vi "Red-Blue Overlay with Select.vi"(7 "RGB IMageRefnum IN":T1, 8 "Blue Channel Refnum":T1, 9 "Enable Blue?":bool, 10 "Red Channel Refnum":T1, 11 "Enable Red?":bool) -> (3 "RGB Image Refnum out OUT":T1)   [LabVIEW 2012]
uses:
  <vilib>/vision/Image Controls.llb/IMAQ Image.ctl
  <vilib>/vision/NI_Vision_Development_Module.lvlib
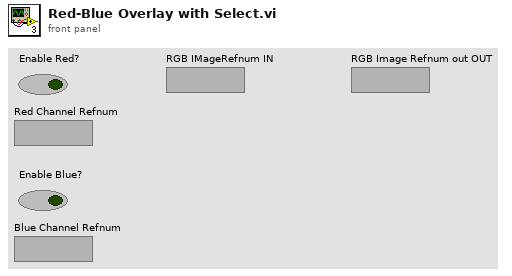
[diagram p1: front panel]
types:
  T1 = typedef "IMAQ Image.ctl" = refnum<image>
  T2 = typedef "Image Type" = u32
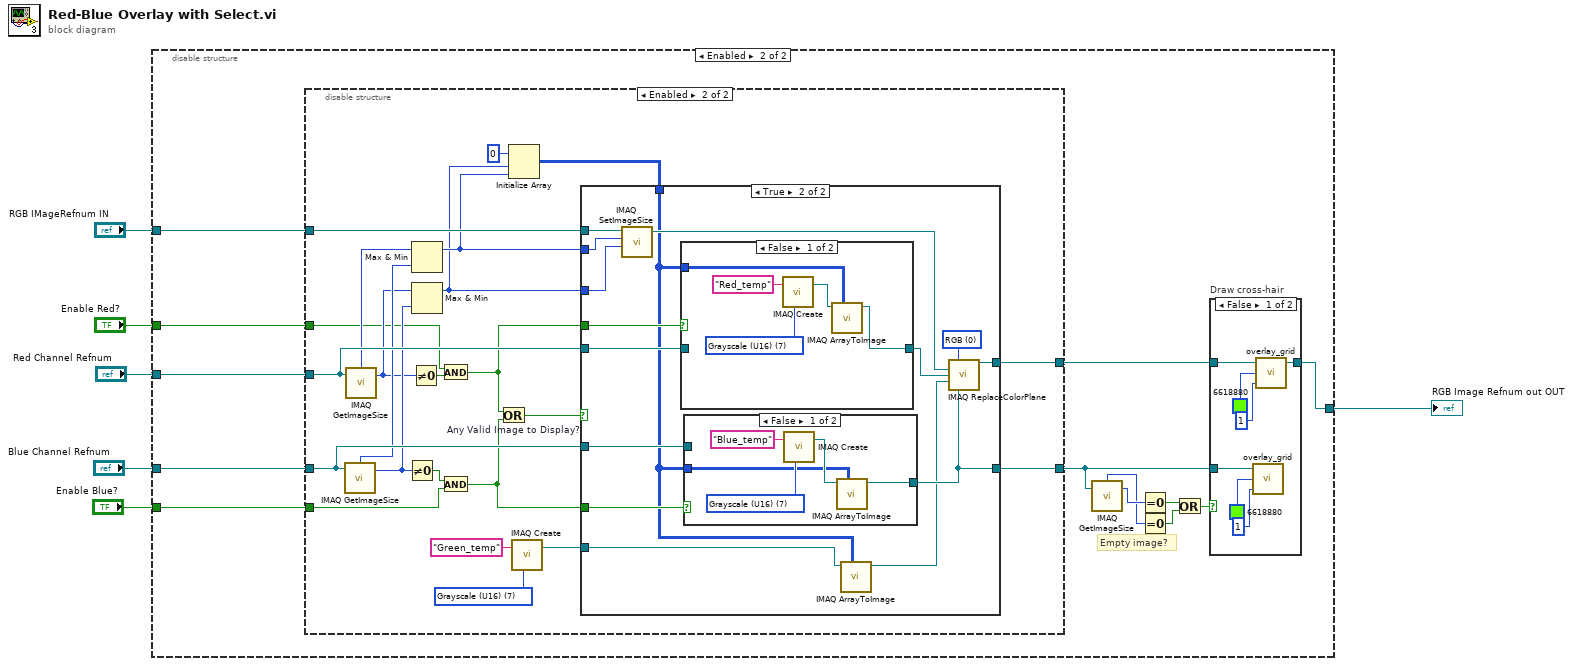
[diagram p0: block diagram]
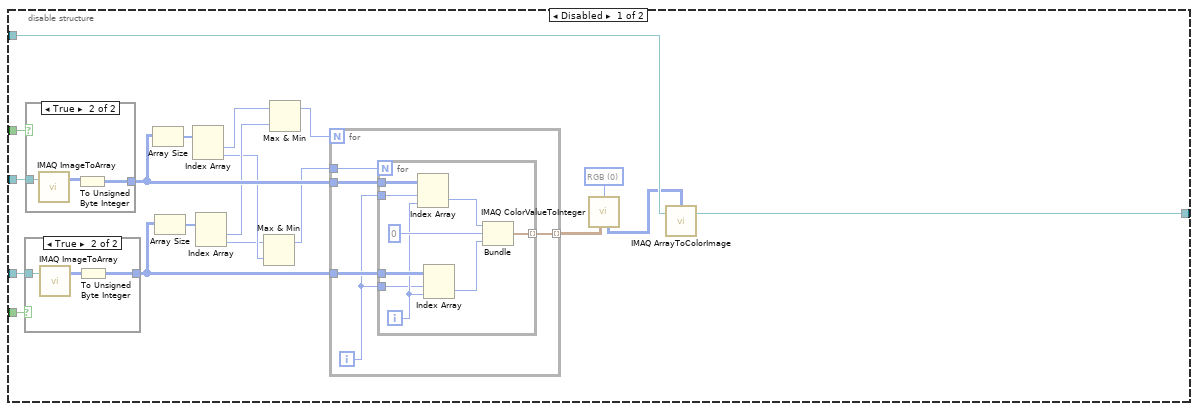
[diagram p2: hidden frame]
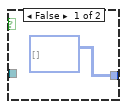
[diagram p3: hidden frame]
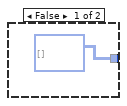
[diagram p4: hidden frame]
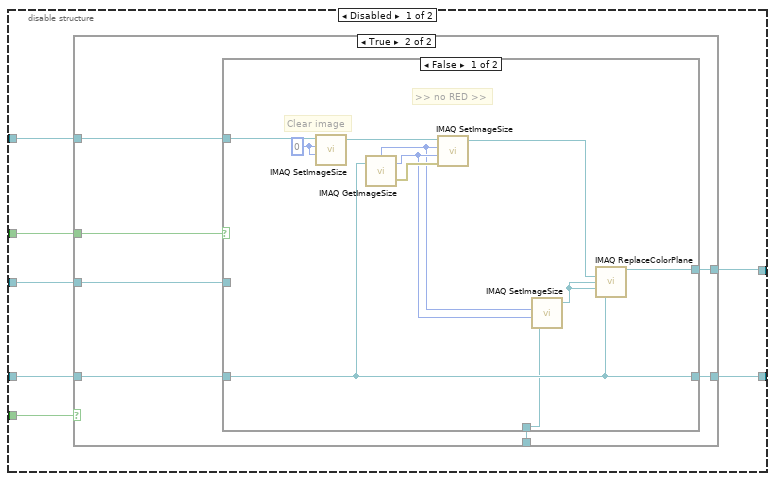
[diagram p5: hidden frame]
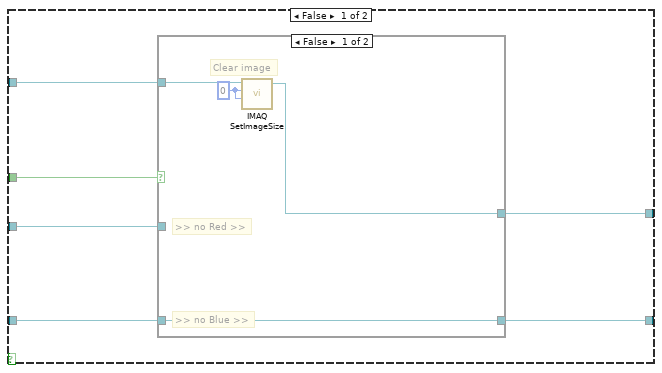
[diagram p6: hidden frame]
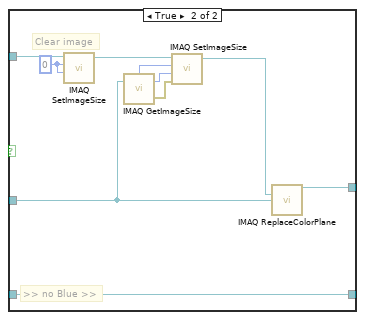
[diagram p7: hidden frame]
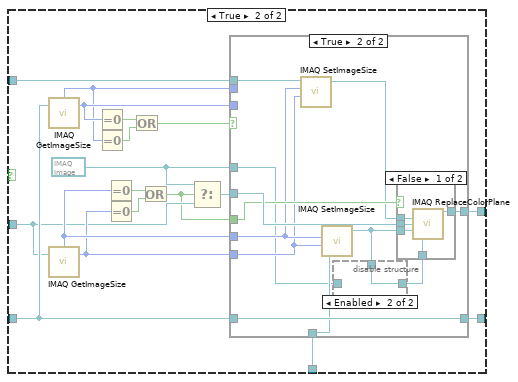
[diagram p8: hidden frame]
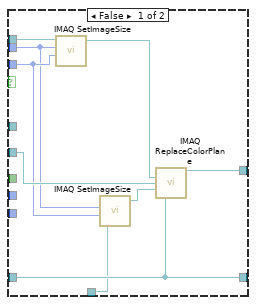
[diagram p9: hidden frame]
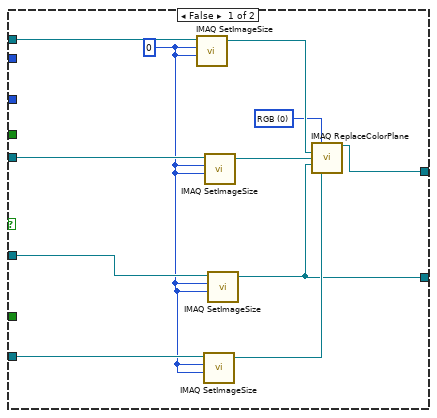
[diagram p12: hidden frame]
diagram:
  n1 = disable-structure shown="Enabled" {
    disable-tunnel: [w25 w48] -> w1
    disable-tunnel: "Blue Channel Refnum" -> [w23 w57]
    disable-tunnel: "Red Channel Refnum" -> [w22 w58]
    disable-tunnel: "RGB IMageRefnum IN" -> [w21 w56]
    disable-tunnel: "Enable Blue?" -> [w18 w59]
    disable-tunnel: "Enable Red?" -> [w17 w60]
    frame Disabled {
      w20 = u16 0 items=["RGB", "HSL", "HSV", "HSI"] ("Color Mode")
      n2 = case shown="True" w18 {
        tunnel: [u8[][] [] w33] -> w16
        tunnel: w23 -> [_ w31]
        frame False {
        }
        frame True {
          n3 = call "IMAQ ImageToArray"("Image"=w31) -> ("Image Pixels (I16)"=w32:i16[][])  [unwired: 3 in, 4 out]
          n4 = To Unsigned Byte Integer(number=w32) -> (unsigned 8bit integer=w33:u8[][])
        }
      }
      n5 = case shown="True" w17 {
        tunnel: [u8[][] [] w29] -> w15
        tunnel: w22 -> [_ w27]
        frame False {
        }
        frame True {
          n6 = call "IMAQ ImageToArray"("Image"=w27) -> ("Image Pixels (I16)"=w28:i16[][])  [unwired: 3 in, 4 out]
          n7 = To Unsigned Byte Integer(number=w28) -> (unsigned 8bit integer=w29:u8[][])
        }
      }
      n8 = Array Size(array=w15) -> (size(s)=w14:i32[])
      n9 = Array Size(array=w16) -> (size(s)=w13:i32[])
      n10 = Index Array(array=w14) -> (element #1=w12:i32, element #2=w9:i32)  [unwired: 2 in]
      n11 = Index Array(array=w13) -> (element #1=w10:i32, element #2=w7:i32)  [unwired: 2 in]
      n12 = Max & Min(x=w7, y=w9) -> (max(x,y)=w8:i32)  [unwired: 1 out]
      n13 = Max & Min(x=w12, y=w10) -> (max(x,y)=w11:i32)  [unwired: 1 out]
      n14 = for {
        N: w11 -> [_]
        tunnel: w16 -> [w35]
        tunnel: w15 -> [w38]
        tunnel: [w37] -> w24 mode=indexing
        tunnel: w8 -> [w36]
        i -> [w34]
        n15 = for {
          N: w36 -> [_]
          tunnel: w38 -> [w44]
          tunnel: [w46] -> w37 mode=indexing
          tunnel: w35 -> [w45]
          tunnel: w34 -> [w42]
          tunnel: w34 -> [w41]
          i -> [w43]
          n16 = Index Array(array=w44, index (row)=w41, index (col)=w43) -> (element=w40:u8)
          n17 = Index Array(array=w45, index (row)=w42, index (col)=w43) -> (element=w39:u8)
          n18 = Bundle(w40, u8 0, w39) -> (w46:cluster{u8, u8, u8})  [unwired: 1 in]
        }
      }
      n19 = call "IMAQ ColorValueToInteger"("2D Color value array"=w24, "Color Mode"=w20) -> ("2D U32 array"=w19:u32[][])  [unwired: 3 in, 3 out]
      n20 = call "IMAQ ArrayToColorImage"("Image Pixels (U32)"=w19, "Image"=w21) -> ("Image Out"=w25:T1)  [unwired: 3 in, 1 out]
    }
    frame Enabled {
      # "Empty image?"
      n21 = disable-structure shown="Enabled" {
        disable-tunnel: w60 -> [w68 w167]
        disable-tunnel: w59 -> [w67 w169]
        disable-tunnel: w58 -> [w66 w175]
        disable-tunnel: w57 -> [w65 w176]
        disable-tunnel: w56 -> [w64 w165]
        disable-tunnel: [w63 w163] -> w52
        disable-tunnel: [w62 w164] -> w49
        frame Disabled {
          n22 = case shown="True" w67 {
            tunnel: w64 -> [w73 w95]
            tunnel: w66 -> [w72 w94]
            tunnel: [w70 w93] -> w62
            tunnel: w68 -> [w74 w92]
            tunnel: w65 -> [w71 w91]
            tunnel: [w69 w90] -> w63
            tunnel: [_ w89] -> w61
            frame False {
              n23 = case shown="False" w74 {
                tunnel: [w76 w88] -> w70
                tunnel: w73 -> [w77 w82]
                tunnel: w72 -> [_ w84]
                tunnel: w71 -> [w75 w80]
                tunnel: [w75 w80] -> w69
                frame False {
                  w78 = 0 ("X Resolution")
                  # "Clear image"
                  # ">> no Blue >>"
                  # ">> no Red >>"
                  n24 = call "IMAQ SetImageSize"("Y Resolution"=w78, "X Resolution"=w78, "Image"=w77) -> ("Image Out"=w76:T1)  [unwired: 2 in, 1 out]
                }
                frame True {
                  w83 = 0 ("X Resolution")
                  # "Clear image"
                  # ">> no Blue >>"
                  n25 = call "IMAQ SetImageSize"("Y Resolution"=w83, "X Resolution"=w83, "Image"=w82) -> ("Image Out"=w81:T1)  [unwired: 2 in, 1 out]
                  n26 = call "IMAQ GetImageSize"("Image"=w84) -> ("Y Resolution"=w86:i32, "X Resolution"=w87:i32, "error out"=w85:errorcluster)  [unwired: 3 in]
                  n27 = call "IMAQ SetImageSize"("error in (no error)"=w85, "Y Resolution"=w86, "X Resolution"=w87, "Image"=w81) -> ("Image Out"=w79:T1)  [unwired: 1 in, 1 out]
                  n28 = call "IMAQ ReplaceColorPlane"("Image Dst"=w79, "Red or Hue Plane"=w84) -> ("Image Dst Out"=w88:T1)  [unwired: 12 in, 1 out]
                }
              }
            }
            frame True {
              n29 = case shown="False" w92 {
                tunnel: w95 -> [w103 w122]
                tunnel: w94 -> [_ w111]
                tunnel: [w106 w124] -> w93
                tunnel: w91 -> [w101 w123]
                tunnel: [w101 w109] -> w90
                tunnel: w89 -> [w99 w107]
                frame False {
                  w104 = 0 ("X Resolution")
                  # "Clear image"
                  # ">> no RED >>"
                  n30 = call "IMAQ SetImageSize"("Y Resolution"=w104, "X Resolution"=w104, "Image"=w103) -> ("Image Out"=w102:T1)  [unwired: 2 in, 1 out]
                  n31 = call "IMAQ GetImageSize"("Image"=w101) -> ("Y Resolution"=w98:i32, "X Resolution"=w97:i32, "error out"=w105:errorcluster)  [unwired: 3 in]
                  n32 = call "IMAQ SetImageSize"("error in (no error)"=w105, "Y Resolution"=w98, "X Resolution"=w97, "Image"=w102) -> ("Image Out"=w100:T1)  [unwired: 1 in, 1 out]
                  n33 = call "IMAQ SetImageSize"("Y Resolution"=w98, "X Resolution"=w97, "Image"=w99) -> ("Image Out"=w96:T1)  [unwired: 2 in, 1 out]
                  n34 = call "IMAQ ReplaceColorPlane"("Image Dst"=w100, "Red or Hue Plane"=w96, "Green or Sat Plane"=w96, "Blue or Luma or Val or Inten Plane"=w101) -> ("Image Dst Out"=w106:T1)  [unwired: 10 in, 1 out]
                }
                frame True {
                  w112 = T1 refnum ("Image Src")
                  n35 = call "IMAQ GetImageSize"("Image"=w123) -> ("Y Resolution"=w121:i32, "X Resolution"=w120:i32)  [unwired: 3 in, 1 out]
                  n36 = call "IMAQ GetImageSize"("Image"=w111) -> ("Y Resolution"=w113:i32, "X Resolution"=w114:i32)  [unwired: 3 in, 1 out]
                  n37 = Equal To 0?(x=w121) -> (x = 0?=w119:bool)
                  n38 = Equal To 0?(x=w120) -> (x = 0?=w118:bool)
                  n39 = Equal To 0?(x=w114) -> (x = 0?=w116:bool)
                  n40 = Equal To 0?(x=w113) -> (x = 0?=w115:bool)
                  n41 = Or(x=w119, y=w118) -> (x .or. y?=w117:bool)
                  n42 = Or(x=w116, y=w115) -> (x .or. y?=w108:bool)
                  n43 = Select(t=w112, s=w108, f=w111) -> (s? t:f=w110:T1)
                  n44 = case shown="True" w117 {
                    tunnel: [w133 w145] -> w124
                    tunnel: w123 -> [w130 w142]
                    tunnel: w122 -> [w132 w144]
                    tunnel: w121 -> [w127 _]
                    tunnel: w120 -> [w126 _]
                    tunnel: w114 -> [_ w138]
                    tunnel: w113 -> [_ w137]
                    tunnel: w112 -> [_ w136]
                    tunnel: w110 -> [w131 w143]
                    tunnel: [w130 w142] -> w109
                    tunnel: w108 -> [_ w141]
                    tunnel: w107 -> [w128 w139]
                    frame False {
                      n45 = call "IMAQ SetImageSize"("Y Resolution"=w127, "X Resolution"=w126, "Image"=w132) -> ("Image Out"=w129:T1)  [unwired: 2 in, 1 out]
                      n46 = call "IMAQ SetImageSize"("Y Resolution"=w127, "X Resolution"=w126, "Image"=w128) -> ("Image Out"=w125:T1)  [unwired: 2 in, 1 out]
                      n47 = call "IMAQ ReplaceColorPlane"("Image Dst"=w129, "Red or Hue Plane"=w131, "Green or Sat Plane"=w125, "Blue or Luma or Val or Inten Plane"=w130) -> ("Image Dst Out"=w133:T1)  [unwired: 10 in, 1 out]
                    }
                    frame True {
                      n48 = call "IMAQ SetImageSize"("Y Resolution"=w137, "X Resolution"=w138, "Image"=w144) -> ("Image Out"=w140:T1)  [unwired: 2 in, 1 out]
                      n49 = call "IMAQ SetImageSize"("Y Resolution"=w137, "X Resolution"=w138, "Image"=w139) -> ("Image Out"=w134:T1)  [unwired: 2 in, 1 out]
                      n50 = disable-structure shown="Enabled" {
                        disable-tunnel: w136 -> [w146 _]
                        disable-tunnel: [w146 w147] -> w135
                        disable-tunnel: w134 -> [_ w147]
                        frame Disabled {
                        }
                        frame Enabled {
                        }
                      }
                      n51 = case shown="False" w141 {
                        tunnel: [w152 w153] -> w145
                        tunnel: w140 -> [w151 w153]
                        tunnel: w135 -> [w150 _]
                        tunnel: w143 -> [w149 _]
                        tunnel: w134 -> [w148 _]
                        frame False {
                          n52 = call "IMAQ ReplaceColorPlane"("Image Dst"=w151, "Red or Hue Plane"=w149, "Green or Sat Plane"=w148, "Blue or Luma or Val or Inten Plane"=w150) -> ("Image Dst Out"=w152:T1)  [unwired: 10 in, 1 out]
                        }
                        frame True {
                        }
                      }
                    }
                  }
                }
              }
            }
          }
        }
        frame Enabled {
          w155 = T2 7 items=["Grayscale (U8)", "Grayscale (I16)", "Grayscale (SGL)", "Complex (CSG)", "RGB (U32)", "HSL (U32)", "RGB (U64)", "Grayscale (U16)"] ("Image Type")
          n53 = call "IMAQ GetImageSize"("Image"=w176) -> ("Y Resolution"=w172:i32, "X Resolution"=w173:i32)  [unwired: 3 in, 1 out]
          n54 = call "IMAQ GetImageSize"("Image"=w175) -> ("Y Resolution"=w171:i32, "X Resolution"=w174:i32)  [unwired: 3 in, 1 out]
          n55 = Not Equal To 0?(x=w172) -> (x != 0?=w170:bool)
          n56 = Not Equal To 0?(x=w171) -> (x != 0?=w168:bool)
          n57 = Max & Min(x=w174, y=w173) -> (max(x,y)=w161:i32)  [unwired: 1 out]
          n58 = Max & Min(x=w171, y=w172) -> (max(x,y)=w160:i32)  [unwired: 1 out]
          n59 = And(x=w167, y=w168) -> (x .and. y?=w158:bool)
          n60 = And(x=w170, y=w169) -> (x .and. y?=w157:bool)
          n61 = Or "Any Valid Image to Display?"(x=w158, y=w157) -> (x .or. y?=w166:bool)
          n62 = Initialize Array(u16 0 ("element"), w160, w161) -> (w159:u16[][])
          n63 = call "IMAQ Create"("Image Name"="Green_temp", "Image Type"=w155) -> ("New Image"=w154:T1)  [unwired: 3 in, 1 out]
          n64 = case shown="True" w166 {
            tunnel: w176 -> [w180 w199]
            tunnel: w175 -> [w185 w202]
            tunnel: w157 -> [_ w201]
            tunnel: w165 -> [w187 w200]
            tunnel: [w181 w196] -> w164
            tunnel: [w178 w192] -> w163
            tunnel: w161 -> [_ w197]
            tunnel: w160 -> [_ w198]
            tunnel: w159 -> [_ w188]
            tunnel: w158 -> [_ w190]
            tunnel: w154 -> [w179 w189]
            frame False {
              w182 = u16 0 items=["RGB", "HSL", "HSV", "HSI"] ("Color Mode")
              w177 = 0 ("X Resolution")
              n65 = call "IMAQ SetImageSize"("Y Resolution"=w177, "X Resolution"=w177, "Image"=w187) -> ("Image Out"=w186:T1)  [unwired: 2 in, 1 out]
              n66 = call "IMAQ SetImageSize"("Y Resolution"=w177, "X Resolution"=w177, "Image"=w179) -> ("Image Out"=w183:T1)  [unwired: 2 in, 1 out]
              n67 = call "IMAQ SetImageSize"("Y Resolution"=w177, "X Resolution"=w177, "Image"=w185) -> ("Image Out"=w184:T1)  [unwired: 2 in, 1 out]
              n68 = call "IMAQ SetImageSize"("Y Resolution"=w177, "X Resolution"=w177, "Image"=w180) -> ("Image Out"=w178:T1)  [unwired: 2 in, 1 out]
              n69 = call "IMAQ ReplaceColorPlane"("Color Mode"=w182, "Image Dst"=w186, "Red or Hue Plane"=w184, "Green or Sat Plane"=w178, "Blue or Luma or Val or Inten Plane"=w183) -> ("Image Dst Out"=w181:T1)  [unwired: 9 in, 1 out]
            }
            frame True {
              w195 = u16 0 items=["RGB", "HSL", "HSV", "HSI"] ("Color Mode")
              n70 = call "IMAQ SetImageSize"("Y Resolution"=w198, "X Resolution"=w197, "Image"=w200) -> ("Image Out"=w194:T1)  [unwired: 2 in, 1 out]
              n71 = case shown="False" w190 {
                tunnel: w202 -> [_ w214]
                tunnel: [w210 w214] -> w193
                tunnel: w188 -> [w209 _]
                frame False {
                  w213 = T2 7 items=["Grayscale (U8)", "Grayscale (I16)", "Grayscale (SGL)", "Complex (CSG)", "RGB (U32)", "HSL (U32)", "RGB (U64)", "Grayscale (U16)"] ("Image Type")
                  n72 = call "IMAQ Create"("Image Name"="Red_temp", "Image Type"=w213) -> ("New Image"=w211:T1)  [unwired: 3 in, 1 out]
                  n73 = call "IMAQ ArrayToImage"("Image Pixels (U16)"=w209, "Image"=w211) -> ("Image Out"=w210:T1)  [unwired: 8 in, 1 out]
                }
                frame True {
                }
              }
              n74 = case shown="False" w201 {
                tunnel: w199 -> [_ w208]
                tunnel: [w204 w208] -> w192
                tunnel: w188 -> [w203 _]
                frame False {
                  w205 = T2 7 items=["Grayscale (U8)", "Grayscale (I16)", "Grayscale (SGL)", "Complex (CSG)", "RGB (U32)", "HSL (U32)", "RGB (U64)", "Grayscale (U16)"] ("Image Type")
                  n75 = call "IMAQ Create"("Image Name"="Blue_temp", "Image Type"=w205) -> ("New Image"=w207:T1)  [unwired: 3 in, 1 out]
                  n76 = call "IMAQ ArrayToImage"("Image Pixels (U16)"=w203, "Image"=w207) -> ("Image Out"=w204:T1)  [unwired: 8 in, 1 out]
                }
                frame True {
                }
              }
              n77 = call "IMAQ ArrayToImage"("Image Pixels (U16)"=w188, "Image"=w189) -> ("Image Out"=w191:T1)  [unwired: 8 in, 1 out]
              n78 = call "IMAQ ReplaceColorPlane"("Color Mode"=w195, "Image Dst"=w194, "Red or Hue Plane"=w193, "Green or Sat Plane"=w191, "Blue or Luma or Val or Inten Plane"=w192) -> ("Image Dst Out"=w196:T1)  [unwired: 9 in, 1 out]
            }
          }
        }
      }
      n79 = call "IMAQ GetImageSize"("Image"=w52) -> ("Y Resolution"=w55:i32, "X Resolution"=w51:i32)  [unwired: 3 in, 1 out]
      n80 = Equal To 0?(x=w55) -> (x = 0?=w54:bool)
      n81 = Equal To 0?(x=w51) -> (x = 0?=w53:bool)
      n82 = Or(x=w54, y=w53) -> (x .or. y?=w50:bool)
      n83 = case "Draw cross-hair" shown="False" w50 {
        tunnel: w52 -> [w219 _]
        tunnel: w49 -> [w216 w222]
        tunnel: [w215 w222] -> w48
        frame False {
          n84 = call "overlay_grid.vi"("no of grid lines"=1, "Color (red)"=u32 6618880 ("Color"), "Image In"=w219) -> ()  [unwired: 2 in, 1 out]
          n85 = call "overlay_grid.vi"("no of grid lines"=1, "Color (red)"=u32 6618880 ("Color"), "Image In"=w216) -> ("Image Out"=w215:T1)  [unwired: 2 in]
        }
        frame True {
        }
      }
    }
  }
  "RGB Image Refnum out OUT" <- w1
